vi "AFG3352X.update services and attribute data for additional services.vi"(0 "i ref in":refnum<vi>, 1 "direction":T2, 2 "Service":enum16{"Mode1", "Mode2", "Burst1", "Burst2"}(ring), 3 "ms timeout (10000)":i32=10000, 4 "value":string, 5 "error in (no error)":errorcluster, 7 "quality":T1=enum."on") -> (14 "i ref out":refnum<vi>, 17 "timed out":bool, 19 "error out":errorcluster)   [LabVIEW 2014, in "AFG3352X.lvlib"]
doc: "Updates the DIM service of a value and updates the attribute data."
uses:
  AFG3352X.lvlib
  CS_Core/CSApplicationBaseClasses/AFGBase/AFGBase.directionType.ctl
  CSlibraries/UtilityLib/UtilityLib.valueStatus.ctl
  CSlibraries-extern/DimLVEvent/LVDimInterface/LVDimInterface.lvlib
  CS_Core/CSSystem/CoreLib/CoreLib.lvlib
  CS_Core/CSApplicationBaseClasses/AFGBase/AFGBase.lvlib
  CSlibraries/UtilityLib/UtilityLib.lvlib
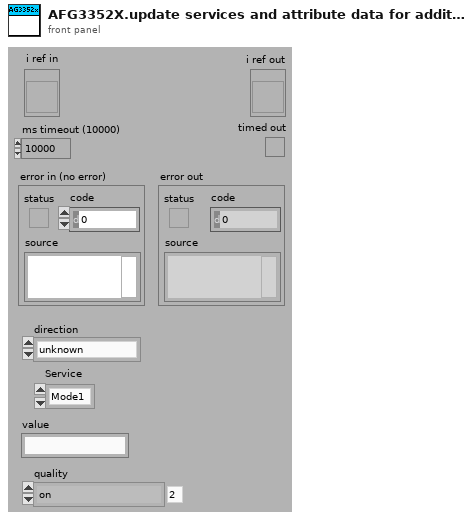
[diagram p1: front panel]
types:
  T1 = typedef "UtilityLib.lvlib/UtilityLib.valueStatus.ctl" = enum16{"no info available", "stand by/off", "on", "warning", "alarm/malfunction", "not implemented", "user action required", "important information", "system default", "control default", "indicator default", "button default"}
  T2 = typedef "AFGBase.lvlib/AFGBase.directionType.ctl" = enum16{"unknown", "update actual value", "update nominal value", "update both"}
  T3 = typedef "AFG3352X.lvlib/AFG3352X.i attribute.ctl" = cluster{"Act2ndValues":cluster{"frequency":dbl, "amplitude":dbl, "phase":dbl, "DCOffset":dbl, "waveformType":T4, "enableOutput":bool, "trigger":i16[], "serviceIDs":cluster{"frequencyID":i32, "amplitudeID":i32, "phaseID":i32, "DCOffsetID":i32, "waveformTypeID":i32, "enableOutputID":i32, "triggerID":i32}, "waveform":cluster{"data":waveform(dbl), "gain":dbl, "offset":dbl, "repetitionRate":dbl, "sampleRate":dbl}}, "Nom2ndValues":cluster{"frequency":dbl, "amplitude":dbl, "phase":dbl, "DCOffset":dbl, "waveformType":T4, "enableOutput":bool, "trigger":i16[], "serviceIDs":cluster{"frequencyID":i32, "amplitudeID":i32, "phaseID":i32, "DCOffsetID":i32, "waveformTypeID":i32, "enableOutputID":i32, "triggerID":i32}, "waveform":cluster{"data":waveform(dbl), "gain":dbl, "offset":dbl, "repetitionRate":dbl, "sampleRate":dbl}}, "DefaultChannel":i32, "ActAddValues":cluster{"Mode1":u16, "serviceIDs":cluster{"Mode1ID":i32, "Mode2ID":i32, "Burst1ID":i32, "Burst2ID":i32}, "Mode2":u16, "Burst1":i32, "Burst2":i32}, "NomAddValues":cluster{"Mode1":u16, "serviceIDs":cluster{"Mode1ID":i32, "Mode2ID":i32, "Burst1ID":i32, "Burst2ID":i32}, "Mode2 2":u16, "Burst1":i32, "Burst2":i32}, "enableBurstMode":bool}
  T4 = typedef "AFGBase.lvlib/AFGBase.waveformType.ctl" = enum16{"sine", "square", "ramp", "pulse", "noise", "DC", "arbitrary", "triangle", "ramp_up", "ramp_down", "amplitude modulation"}
  T5 = cluster{"Mode1":u16, "serviceIDs":cluster{"Mode1ID":i32, "Mode2ID":i32, "Burst1ID":i32, "Burst2ID":i32}, "Mode2":u16, "Burst1":i32, "Burst2":i32}
  T6 = cluster{"Mode1":u16, "serviceIDs":cluster{"Mode1ID":i32, "Mode2ID":i32, "Burst1ID":i32, "Burst2ID":i32}, "Mode2 2":u16, "Burst1":i32, "Burst2":i32}
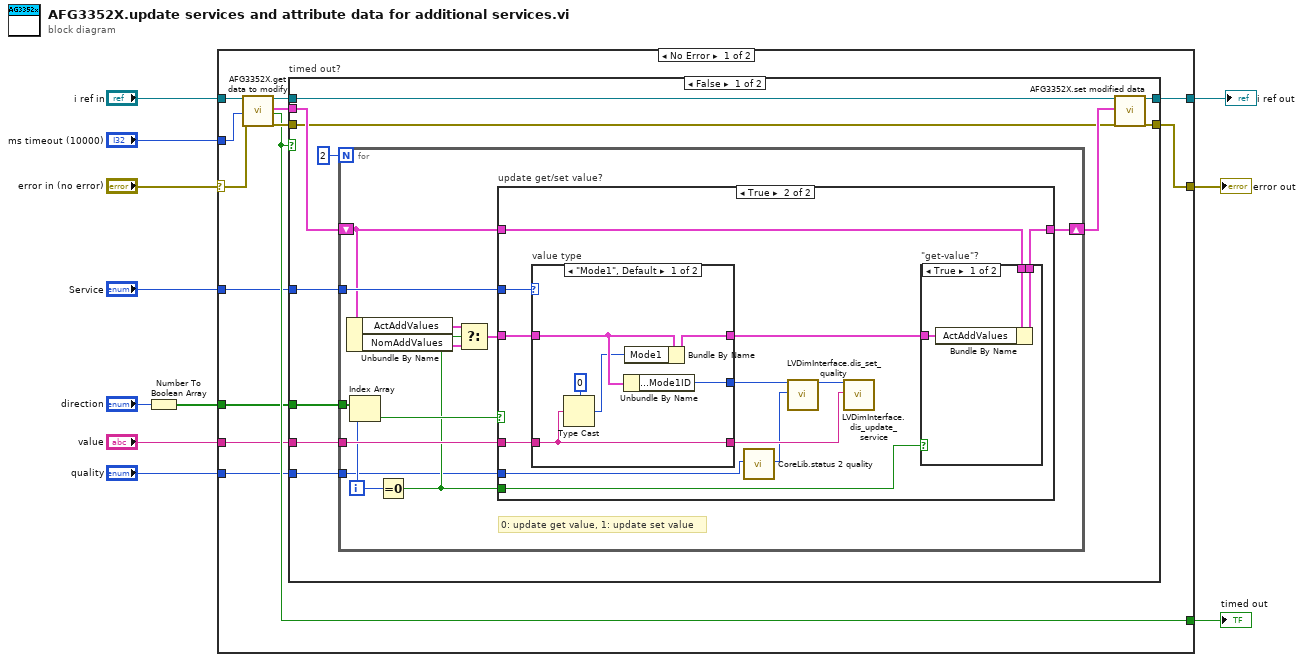
[diagram p0: block diagram]
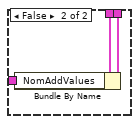
[diagram p3: hidden frame]
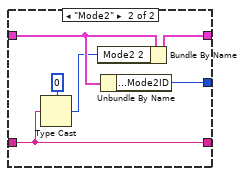
[diagram p4: hidden frame]
diagram:
  n1 = Number To Boolean Array(number="direction") -> (Boolean array=w6:bool[])
  n2 = case shown="No Error" "error in (no error)" {
    selector: "error in (no error)" -> [w22 w82]
    tunnel: [w18 w82] -> w10
    tunnel: "i ref in" -> [w24 w81]
    tunnel: [w20 w81] -> w2
    tunnel: "ms timeout (10000)" -> [w23 _]
    tunnel: [w17 _] -> w8
    tunnel: w6 -> [w15 _]
    tunnel: "Service" -> [w14 _]
    tunnel: "value" -> [w13 _]
    tunnel: "quality" -> [w12 _]
    frame No Error {
      n3 = call "AFG3352X.get data to modify.vi"("i ref in"=w24, "ms timeout (10000)"=w23, "error in (no error)"=w22) -> ("i ref out"=w21:refnum<vi>, "i attribute"=w16:T3, "timed out"=w17:bool, "error out"=w19:errorcluster)  [unwired: 13 in]
      n4 = case "timed out?" shown="False" w17 {
        tunnel: w21 -> [w33 w80]
        tunnel: [w35 w80] -> w20
        tunnel: w19 -> [w26 w79]
        tunnel: [w34 w79] -> w18
        tunnel: w16 -> [w30 _]
        tunnel: w15 -> [w31 _]
        tunnel: w14 -> [w29 _]
        tunnel: w13 -> [w28 _]
        tunnel: w12 -> [w25 _]
        frame False {
          n5 = for {
            N: 2 -> [_]
            tunnel: w31 -> [w47]
            tunnel: w29 -> [w45]
            tunnel: w28 -> [w44]
            tunnel: w25 -> [w36]
            shift-right: [w37] -> w27
            shift-left: w30 -> [w39]
            i -> [w43]
            # "0: update get value, 1: update set value"
            n6 = Unbundle By Name(w39) -> ("ActAddValues"=w42:T5, "NomAddValues"=w41:T6)
            n7 = Index Array(array=w47, index=w43) -> (element=w46:bool)
            n8 = Equal To 0?(x=w43) -> (x = 0?=w38:bool)
            n9 = Select(t=w42, s=w38, f=w41) -> (s? t:f=w40:T6)
            n10 = case "update get/set value?" shown="True" w46 {
              tunnel: w45 -> [_ w60]
              tunnel: w44 -> [_ w57]
              tunnel: w40 -> [_ w58]
              tunnel: w39 -> [w48 w56]
              tunnel: w38 -> [_ w54]
              tunnel: [w48 w53] -> w37
              tunnel: w36 -> [_ w52]
              frame False {
              }
              frame True {
                n11 = case "value type" shown="\"Mode1\", Default" w60 {
                  tunnel: w58 -> [w71 w77]
                  tunnel: [w72 w78] -> w50
                  tunnel: [w67 w73] -> w59
                  tunnel: w57 -> [w67 w73]
                  tunnel: [w70 w76] -> w55
                  frame "Mode1", Default {
                    n12 = Type Cast(type=0, x=w67) -> (*(type *) &x=w68:i32)
                    n13 = Unbundle By Name(w71) -> ("serviceIDs.Mode1ID"=w72:i32)
                    n14 = Bundle By Name(cluster=w71, "Mode1"=w68) -> (w70:T6)
                  }
                  frame "Mode2" {
                    n15 = Type Cast(type=0, x=w73) -> (*(type *) &x=w74:i32)
                    n16 = Bundle By Name(cluster=w77, "Mode2 2"=w74) -> (w76:T6)
                    n17 = Unbundle By Name(w77) -> ("serviceIDs.Mode2ID"=w78:i32)
                  }
                }
                n18 = call "CoreLib.status 2 quality.vi"("valueStatus"=w52) -> ("quality"=w51:i32)  [unwired: 18 in]
                n19 = call "LVDimInterface.dis_set_quality.vi"("my_serviceID"=w50, "quality"=w51) -> ("my_serviceID (out)"=w49:i32)  [unwired: 16 in, 1 out]
                n20 = call "LVDimInterface.dis_update_service.vi"("my_serviceID"=w49, "data"=w59) -> ()  [unwired: 15 in, 3 out]
                n21 = case "\"get-value\"?" shown="True" w54 {
                  tunnel: w56 -> [w63 w66]
                  tunnel: w55 -> [w62 w65]
                  tunnel: [w61 w64] -> w53
                  frame True {
                    n22 = Bundle By Name(cluster=w63, "ActAddValues"=w62) -> (w61:T3)
                  }
                  frame False {
                    n23 = Bundle By Name(cluster=w66, "NomAddValues"=w65) -> (w64:T3)
                  }
                }
              }
            }
          }
          n24 = call "AFG3352X.set modified data.vi"("i ref in"=w33, "i attribute"=w27, "error in (no error)"=w26) -> ("i ref out"=w35:refnum<vi>, "error out"=w34:errorcluster)  [unwired: 15 in]
        }
        frame True {
        }
      }
    }
    frame Error {
    }
  }
  "error out" <- w10
  "timed out" <- w8
  "i ref out" <- w2
